vi "PMTs Control module.vi"(8 "Error In":errorcluster, 9 "Cancelled":bool, 11 "Function":T1) -> (0 "Error Out":errorcluster)   [LabVIEW 2017]
uses:
  Typedefs/PMT control functions.ctl
  Global Variables/gl_UI Ctrl Refs.vi
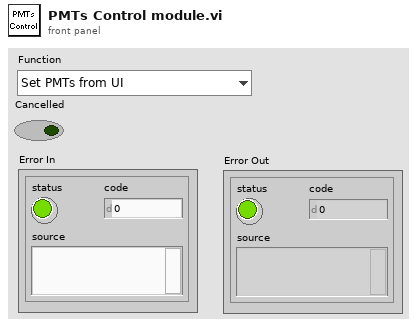
[diagram p1: front panel]
types:
  T1 = typedef "PMT control functions.ctl" = enum16{"Set PMTs from UI", "Reset PMTs"}
  T2 = typedef "UI ctrl refs cluster.ctl" = cluster{"Top level VI path":path, "Top level VI ref":refnum<vi>, "User menu ref":refnum<k9>, "Sub Panel control":refnum<vi>, "Imaging Param Tab":refnum<vi>, "Occurrence-Start drivers":refnum<k4>, "Occurrence-Speed logging initialised":refnum<k4>, "Occurrence-XYZ stage initialised":refnum<k4>, "Exit button":refnum<vi>, "Status ind":refnum<vi>, "Set as origin":refnum<vi>, "Speed Logging":refnum<vi>, "Time Lapse":refnum<vi>, "Live Imaging":refnum<vi>, "AOL Z Stack":refnum<vi>, "Motor Z Stack":refnum<vi>, "Funct Acq button":refnum<vi>, "Hard Shutter":refnum<vi>, "Virtual Shutter":refnum<vi>, "Laser Power":refnum<vi>, "AOL Mode":refnum<vi>, "Frame Size":refnum<vi>, "Field of View":refnum<vi>, "Dwell Time":refnum<vi>, "Zoom":refnum<vi>, "AOL Z":refnum<vi>, "Objective":refnum<vi>, "Axis":refnum<vi>, "Paths & Names":refnum<vi>, "Experiment folder path (ind.)":refnum<vi>, "Last State (Ind.)":refnum<vi>, "Laser wavelength ind (nm)":refnum<vi>, "Averages":refnum<vi>, "Angle (degrees)":refnum<vi>, "X centre":refnum<vi>, "Y centre":refnum<vi>, "Plane Mode":refnum<vi>, "# Planes":refnum<vi>, "Z Start":refnum<vi>, "Z Stop":refnum<vi>, "Z Step":refnum<vi>, "PMT 1":refnum<vi>, "PMT 2":refnum<vi>, "Stage XYZ Position":refnum<vi>, "Pockels@Z Start":refnum<vi>, "Pockels@Z Stop":refnum<vi>, "Obtain Z Start":refnum<vi>, "Obtain Z Stop":refnum<vi>, "Live stim.trig.period":refnum<vi>, "Live stim.trig.enable":refnum<vi>, "Movement Correction":refnum<vi>, "Load Reference Image":refnum<vi>, "XY Stage Move":refnum<vi>, "MovCor Cluster":refnum<vi>, "RefDAQParam":refnum<vi>, "Funct. Acq. Pockels Modulation":refnum<vi>, "Background MovCor":refnum<vi>, "Ref Laser Power":refnum<vi>, "Enable Video Recording":refnum<vi>, "Video Record-Live Imaging":refnum<vi>, "Video Record-Funct acq":refnum<vi>, "Reference Source":refnum<vi>, "AOL Z-stack Chirps Ready (ind)":refnum<vi>, "Target time between mov.cor. ref triggers (ms)":refnum<vi>, "Funct. Acq. Ref frame save":refnum<vi>, "Tracking button":refnum<vi>, "Show ref plots window":refnum<vi>, "Center freq ind (nm)":refnum<vi>, "Pickup mode (ind)":refnum<vi>, "Logging queue (ind)":refnum<vi>, "Back aperture power (ind.)":refnum<vi>, "Power after objective (ind.)":refnum<vi>, "Switch user":refnum<vi>}
  T3 = typedef "PMT control knob.ctl" = u16
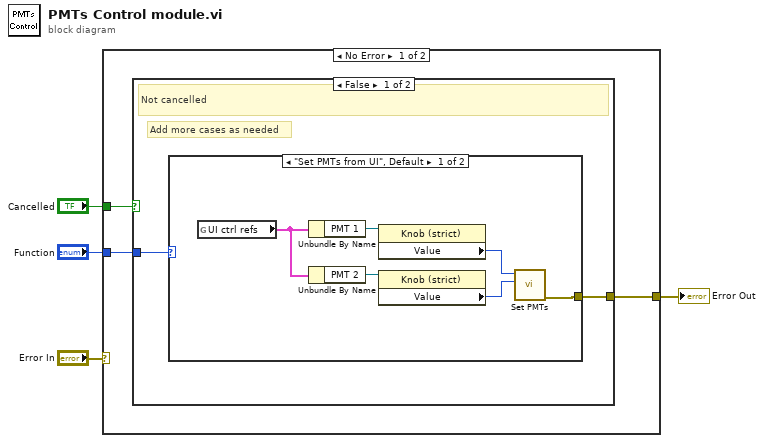
[diagram p0: block diagram]
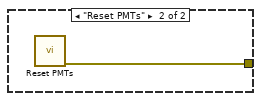
[diagram p2: hidden frame]
diagram:
  n1 = case shown="No Error" "Error In" {
    selector: "Error In" -> [_ w17]
    tunnel: "Function" -> [w7 _]
    tunnel: [w6 w17] -> w3
    tunnel: "Cancelled" -> [w5 _]
    frame No Error {
      n2 = case shown="False" w5 {
        tunnel: w7 -> [w9 _]
        tunnel: [w8 _] -> w6
        frame False {
          # "Add more cases as needed"
          # "Not cancelled"
          n3 = case shown="\"Set PMTs from UI\", Default" w9 {
            tunnel: [w10 w16] -> w8
            frame "Set PMTs from UI", Default {
              n4 = global read "gl_UI Ctrl Refs.vi" "UI ctrl refs"() -> (w15:T2)
              n5 = Unbundle By Name(w15) -> ("PMT 1"=w13:refnum<vi>)
              n6 = Unbundle By Name(w15) -> ("PMT 2"=w14:refnum<vi>)
              n7 = property class="Knob (strict)"(reference=w13) -> ("Value"=w12:T3)  [unwired: 1 in, 2 out]
              n8 = property class="Knob (strict)"(reference=w14) -> ("Value"=w11:T3)  [unwired: 1 in, 2 out]
              n9 = call "Set PMTs.vi"("PMT 2"=w11, "PMT 1"=w12) -> ("Error Out"=w10:errorcluster)  [unwired: 9 in]
            }
            frame "Reset PMTs" {
              n10 = call "Reset PMTs.vi"() -> ("Error Out"=w16:errorcluster)  [unwired: 11 in]
            }
          }
        }
        frame True {
          # "Cancelled"
        }
      }
    }
    frame Error {
    }
  }
  "Error Out" <- w3
